vi "Update Cycle States.vi"(8 "error in (no error)":errorcluster, 10 "Cycle State Message":string, 11 "Main_UI in":refnum<class "Main_UI.lvclass">) -> (0 "error out":errorcluster, 3 "Main_UI out":refnum<class "Main_UI.lvclass">)   [LabVIEW 2020, in "Main_UI.lvlib" / "Main_UI.lvclass"]
uses:
  Main_UI.lvclass
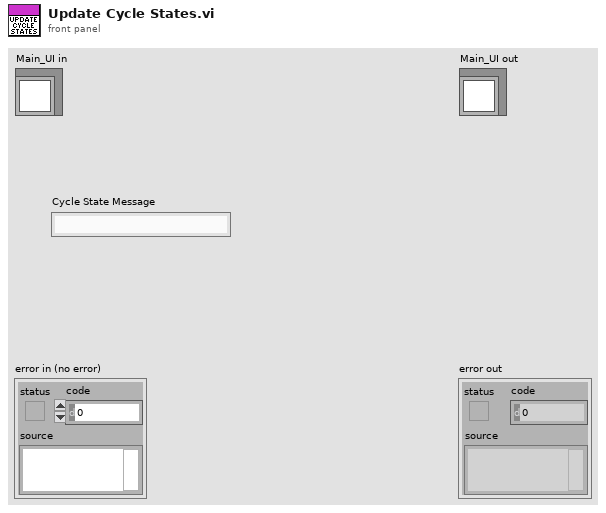
[diagram p1: front panel]
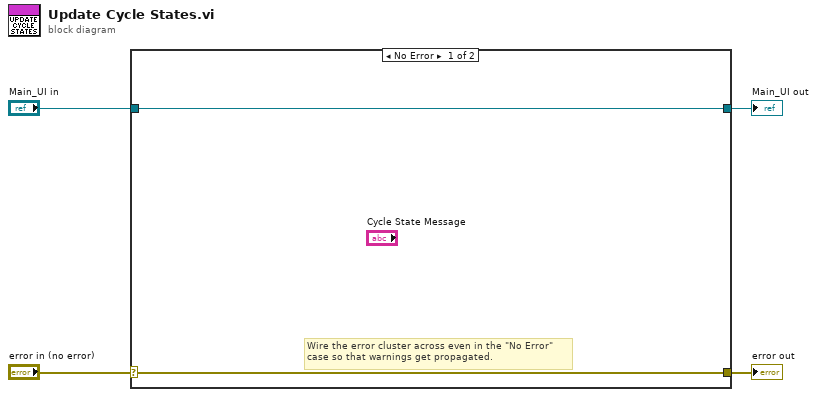
[diagram p0: block diagram]
diagram:
  n1 = case shown="No Error" "error in (no error)" {
    selector: "error in (no error)" -> [w5 w8]
    tunnel: [w5 w8] -> w3
    tunnel: [w6 w7] -> w1
    tunnel: "Main_UI in" -> [w6 w7]
    frame No Error {
      # "Wire the error cluster across even in the \"No Error\"\ncase so that warnings get propagated."
    }
    frame Error {
    }
  }
  "error out" <- w3
  "Main_UI out" <- w1
